vi "Image Histogram v2.vi"(0 "Image in":T2, 7 "Max Percentile (0-100)":dbl min=0.0 max=100.0, 9 "Min Percentile (0-100)":dbl min=0.0 max=100.0, 11 "Error In":errorcluster, 12 "Number of Classes (256)":i32=256) -> (4 "Image Histogram":cluster{"X Array":dbl[], "Y Array":dbl[]}, 6 "Image Statistics":T1, 8 "Highest Percentile Value":dbl, 10 "Lowest Percentile Value":dbl, 13 "Y Resolution":i32, 14 "X Resolution":i32, 15 "Error Out":errorcluster)   [LabVIEW 2021, in "Image.lvlib"]
uses:
  Image.lvlib
  <vilib>/vision/Image Controls.llb/IMAQ Image.ctl
  Image Statistics.ctl
  Histograms/Linear Histogram Options.ctl
  Histograms/Histogram Bin Option.ctl
  Histograms/Histogram Bin Position.ctl
  c276fd47-d12c-459f-8fea-3c7eaaa4422e.vi
  7f1cc798-c783-47f9-b164-3d36a8ec5120.vi
  4fd4f1ad-5643-47d1-b4fe-3f02ed4056f4.vi
  a02382de-93e2-42fe-ad6b-54257930eea8.vi
  a02382de-93e2-42fe-ad6b-54257930eea8.vi/e021cd17-e000-4244-b7f4-ec50548bdfcb.vi
  a02382de-93e2-42fe-ad6b-54257930eea8.vi/b1828c6e-eb0a-43e9-a724-8b596c52e435.vi
  a02382de-93e2-42fe-ad6b-54257930eea8.vi/7a6138ed-c001-4311-b538-9ba42ae7c7b1.vi
  a02382de-93e2-42fe-ad6b-54257930eea8.vi/52c6b4fa-501b-4af0-803b-8bab516ca5d3.vi
  a02382de-93e2-42fe-ad6b-54257930eea8.vi/d7237e10-35ab-4bcb-a0c6-4883c3f4c990.vi
  a02382de-93e2-42fe-ad6b-54257930eea8.vi/5fb5dd96-3b97-4592-ba56-58181c8e7105.vi
  a02382de-93e2-42fe-ad6b-54257930eea8.vi/8e13a849-a393-4484-9968-4af7b25c38d7.vi
  <vilib>/Utility/error.llb/Error Cluster From Error Code.vi
  Time/High Resolution Timing.vi
  <userlib>/_OpenG.lib/array/array.llb/Filter 1D Array__ogtk.vi
  <userlib>/_OpenG.lib/array/array.llb/Filter 1D Array (SGL)__ogtk.vi
  <userlib>/_OpenG.lib/array/array.llb/Delete Elements from Array__ogtk.vi
  <userlib>/_OpenG.lib/array/array.llb/Delete Elements from 1D Array (DBL)__ogtk.vi
  <vilib>/ErrorRing/Error Ring.xnode
  Histograms/Histogram Window.lvlib
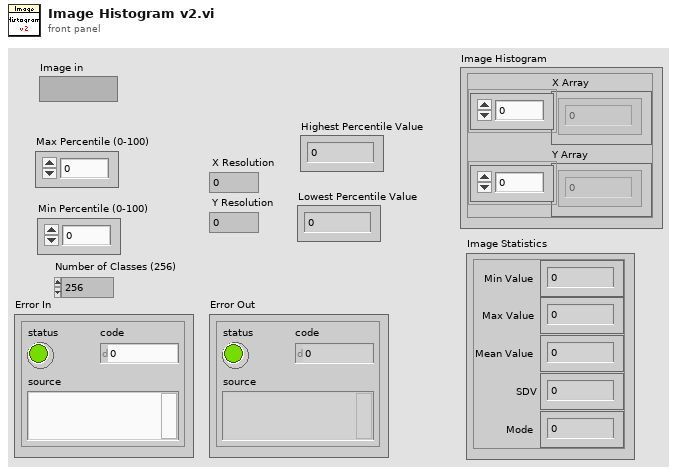
[diagram p1: front panel]
types:
  T1 = typedef "Image.lvlib/Image Statistics.ctl" = cluster{"Min Value":dbl, "Max Value":dbl, "Mean Value":dbl, "SDV":dbl, "Mode":dbl}
  T2 = typedef "IMAQ Image.ctl" = refnum<image>
  T3 = typedef "Histogram Window.lvlib/Linear Histogram Options.ctl" = cluster{"Bin Size":dbl, "Bin Number":i32, "Bin Option":T4, "Min Value":dbl, "Max Value":dbl, "Filter NaN & Infinite Values":bool, "Frequency Plot":bool, "Align Bins":bool, "Bin Location":T5, "Project Outside Values":bool, "Max Histogram Size":i32}
  T4 = typedef "Histogram Window.lvlib/Histogram Bin Option.ctl" = enum32{"Bin Number", "Bin Size"}
  T5 = typedef "Histogram Window.lvlib/Histogram Bin Position.ctl" = enum16{"Left", "Center", "Right"}
  T6 = typedef "Image Type" = u32
  T7 = typedef "Arrays.lvlib/Array Statistics.ctl" = cluster{"Mean":dbl, "Standard Deviation":dbl, "Max":dbl, "Min":dbl}
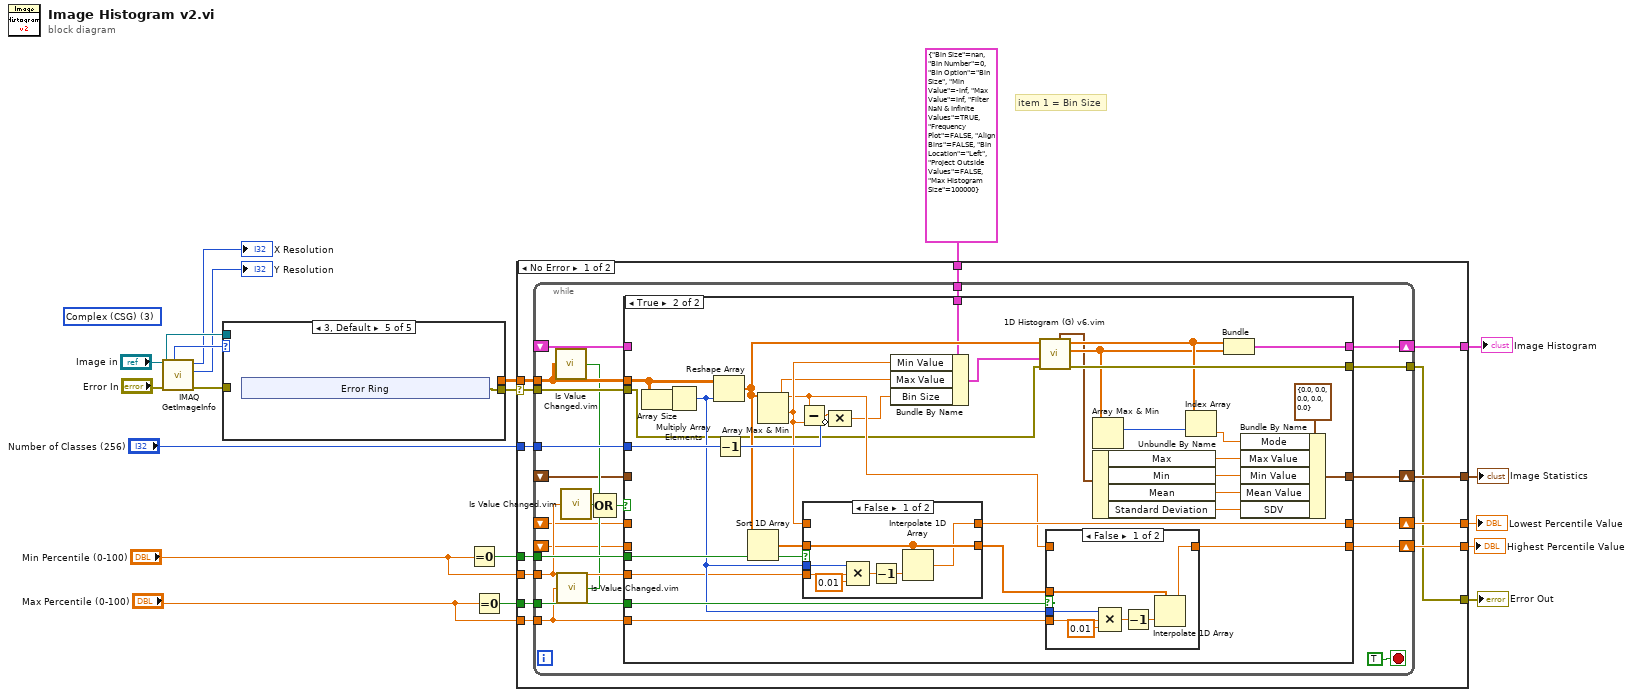
[diagram p0: block diagram]
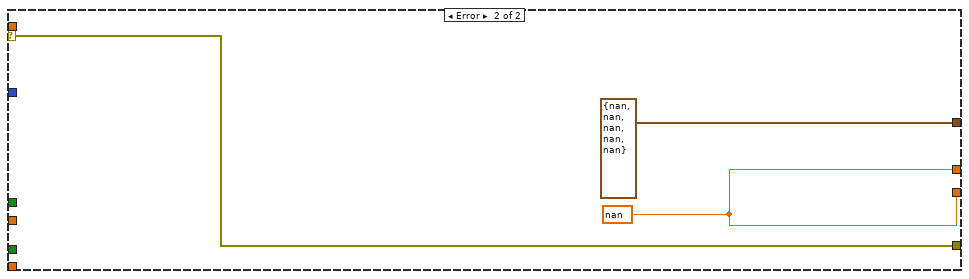
[diagram p5: hidden frame]
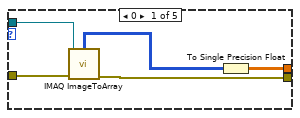
[diagram p6: hidden frame]
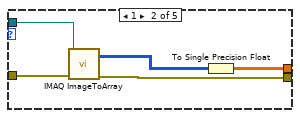
[diagram p7: hidden frame]
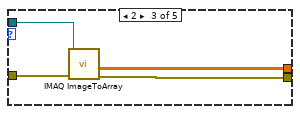
[diagram p8: hidden frame]
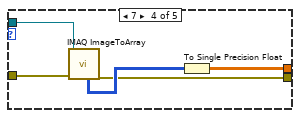
[diagram p9: hidden frame]
diagram:
  (unwired) T6 3 items=["Grayscale (U8)", "Grayscale (I16)", "Grayscale (SGL)", "Complex (CSG)", "RGB (U32)", "HSL (U32)", "RGB (U64)", "Grayscale (U16)"] ("Image Type")
  # "item 1 = Bin Size"
  n1 = call "IMAQ GetImageInfo"("error in (no error)"="Error In", "Image"="Image in") -> ("error out"=w16:errorcluster, "Y Resolution"=→"Y Resolution":i32, "X Resolution"=→"X Resolution":i32, "Image Type"=w15:T6)  [unwired: 2 in, 4 out]
  n2 = case shown="3, Default" w15 {
    tunnel: "Image in" -> [w24 w29 w33 w38 _]
    tunnel: w16 -> [w23 w28 w32 w37 _]
    tunnel: [w20 w25 w31 w34 _] -> w12
    tunnel: [w21 w26 w30 w35 w39] -> w11
    frame 0 {
      n3 = call "IMAQ ImageToArray"("error in (no error)"=w23, "Image"=w24) -> ("error out"=w21:errorcluster, "Image Pixels (U8)"=w22:u8[][])  [unwired: 2 in, 3 out]
      n4 = To Single Precision Float(number=w22) -> (single precision float=w20:sgl[][])
    }
    frame 1 {
      n5 = call "IMAQ ImageToArray"("error in (no error)"=w28, "Image"=w29) -> ("error out"=w26:errorcluster, "Image Pixels (I16)"=w27:i16[][])  [unwired: 2 in, 3 out]
      n6 = To Single Precision Float(number=w27) -> (single precision float=w25:sgl[][])
    }
    frame 2 {
      n7 = call "IMAQ ImageToArray"("error in (no error)"=w32, "Image"=w33) -> ("Image Pixels (Float)"=w31:sgl[][], "error out"=w30:errorcluster)  [unwired: 2 in, 3 out]
    }
    frame 7 {
      n8 = call "IMAQ ImageToArray"("error in (no error)"=w37, "Image"=w38) -> ("Image Pixels (U16)"=w36:u16[][], "error out"=w35:errorcluster)  [unwired: 2 in, 3 out]
      n9 = To Single Precision Float(number=w36) -> (single precision float=w34:sgl[][])
    }
    frame 3, Default {
      n10 = xnode "Error Ring"() -> ("error out"=w39:errorcluster)
    }
  }
  n11 = Equal To 0?(x="Min Percentile (0-100)") -> (x = 0?=w10:bool)
  n12 = Equal To 0?(x="Max Percentile (0-100)") -> (x = 0?=w6:bool)
  n13 = case shown="No Error" w11 {
    selector: w11 -> [w46 w137]
    tunnel: [w56 _] -> w14
    tunnel: w12 -> [w55 _]
    tunnel: "Number of Classes (256)" -> [w54 _]
    tunnel: [w45 w137] -> w13
    tunnel: w10 -> [w53 _]
    tunnel: "Min Percentile (0-100)" -> [w52 _]
    tunnel: [w51 w136] -> w8
    tunnel: [w50 w136] -> w7
    tunnel: w6 -> [w49 _]
    tunnel: "Max Percentile (0-100)" -> [w48 _]
    tunnel: [w47 T1 {"Min Value"=nan, "Max Value"=nan, "Mean Value"=nan, "SDV"=nan, "Mode"=nan} ("Image Statistics")] -> w4
    tunnel: T3 {"Bin Size"=nan, "Bin Number"=0, "Bin Option"=enum."Bin Size", "Min Value"=-inf, "Max Value"=inf, "Filter NaN & Infinite Values"=TRUE, "Frequency Plot"=FALSE, "Align Bins"=FALSE, "Bin Location"=enum."Left", "Project Outside Values"=FALSE, "Max Histogram Size"=100000} ("Histogram Options") -> [w44 _]
    frame No Error {
      n14 = while {
        tunnel: w55 -> [w67]
        tunnel: w54 -> [w77]
        tunnel: w53 -> [w76]
        tunnel: w52 -> [w66]
        tunnel: w49 -> [w73]
        tunnel: w48 -> [w65]
        tunnel: w44 -> [w70]
        tunnel: w46 -> [w69]
        tunnel: [w71] -> w45
        shift-right: [w78] -> w56
        shift-left: _ -> [w60]
        shift-right: [w75] -> w51
        shift-left: _ -> [w59]
        shift-right: [w74] -> w50
        shift-left: _ -> [w58]
        shift-right: [w72] -> w47
        shift-left: _ -> [w57]
        stop <- TRUE stop-if-true
        n15 = call "Is Value Changed.vim"("value"=w67) -> ("changed or first call?"=w63:bool)
        n16 = call "Is Value Changed.vim"("value"=w65) -> ("changed or first call?"=w62:bool)
        n17 = call "Is Value Changed.vim"("value"=w66) -> ("changed or first call?"=w64:bool)
        n18 = Compound Arithmetic op=OR(w63, w64, w62) -> (w61:bool)
        n19 = case shown="True" w61 {
          tunnel: [w82 w117] -> w78
          tunnel: w77 -> [_ w114]
          tunnel: w76 -> [_ w111]
          tunnel: [w81 w110] -> w75
          tunnel: [w80 w109] -> w74
          tunnel: w73 -> [_ w107]
          tunnel: [w79 w99] -> w72
          tunnel: [w83 w96] -> w71
          tunnel: w70 -> [_ w93]
          tunnel: w69 -> [w83 w87]
          tunnel: w67 -> [_ w86]
          tunnel: w66 -> [_ w85]
          tunnel: w65 -> [_ w84]
          tunnel: w60 -> [w82 _]
          tunnel: w59 -> [w81 _]
          tunnel: w58 -> [w80 _]
          tunnel: w57 -> [w79 _]
          frame False {
            # "no need to repeat the calculations"
          }
          frame True {
            n20 = Array Size(array=w86) -> (size(s)=w116:i32[])
            n21 = Multiply Array Elements(1:w116) -> (0:w106:i32)
            n22 = Reshape Array(w86, w106) -> (w97:sgl[])
            n23 = Decrement(x=w114) -> (x-1=w113:i32)
            n24 = Sort 1D Array(array=w97) -> (sorted array=w105:sgl[])
            n25 = Array Max & Min(array=w97) -> (max value=w90:sgl, min value=w91:sgl)  [unwired: 2 out]
            n26 = Subtract(x=w90, y=w91) -> (x-y=w115:sgl)
            n27 = case shown="False" w111 {
              tunnel: w105 -> [w128 w134]
              tunnel: [w128 w134] -> w108
              tunnel: w85 -> [w131 _]
              tunnel: w106 -> [w132 _]
              tunnel: w91 -> [_ w133]
              tunnel: [w127 w133] -> w110
              frame False {
                n28 = Compound Arithmetic op=MULTIPLY(w132, w131, 0.01 ("value")) -> (w129:dbl)
                n29 = Decrement(x=w129) -> (x-1=w126:dbl)
                n30 = Interpolate 1D Array(1:w126, 2:w128) -> (0:w127:sgl)
              }
              frame True {
              }
            }
            n31 = Compound Arithmetic op=MULTIPLY(w115, invert w113) -> (w89:dbl)
            n32 = Bundle By Name(cluster=w93, "Min Value"=w91, "Max Value"=w90, "Bin Size"=w89) -> (w92:T3)
            n33 = call "1D Histogram (G) v6.vim"("Error In"=w87, "Histogram Options"=w92, "Array"=w97) -> ("Error Out"=w96:errorcluster, "Histogram"=w94:dbl[], "Axis"=w95:dbl[], "Array Statistics"=w88:T7)  [unwired: 2 in, 3 out]
            n34 = case shown="False" w107 {
              tunnel: w108 -> [w120 _]
              tunnel: w84 -> [w123 _]
              tunnel: w106 -> [w124 _]
              tunnel: w90 -> [_ w125]
              tunnel: [w119 w125] -> w109
              frame False {
                n35 = Compound Arithmetic op=MULTIPLY(w124, w123, 0.01 ("value")) -> (w121:dbl)
                n36 = Decrement(x=w121) -> (x-1=w118:dbl)
                n37 = Interpolate 1D Array(1:w118, 2:w120) -> (0:w119:sgl)
              }
              frame True {
              }
            }
            n38 = Array Max & Min(array=w94) -> (max index (indices)=w112:i32)  [unwired: 3 out]
            n39 = Unbundle By Name(w88) -> ("Max"=w103:dbl, "Min"=w102:dbl, "Mean"=w101:dbl, "Standard Deviation"=w100:dbl)
            n40 = Index Array(array=w95, index=w112) -> (element=w104:dbl)
            n41 = Bundle("Axis"=w95, "Histogram"=w94) -> (w117:cluster{"Axis":dbl[], "Histogram":dbl[]})  [unwired: 1 in]
            n42 = Bundle By Name(cluster=T1 {"Min Value"=0.0, "Max Value"=0.0, "Mean Value"=0.0, "SDV"=0.0, "Mode"=0.0} ("Image Statistics"), "Mode"=w104, "Max Value"=w103, "Min Value"=w102, "Mean Value"=w101, "SDV"=w100) -> (w99:T1)
          }
        }
      }
    }
    frame Error {
      w136 = nan ("Numeric")
    }
  }
  "Error Out" <- w13
  "Image Histogram" <- w14
  "Image Statistics" <- w4
  "Lowest Percentile Value" <- w8
  "Highest Percentile Value" <- w7
